vi "TankDrive.vi"(0 "RobotDriveDevRef":T2={"DevStatus"={"status"=FALSE, "code"=0, "source"=""}, "Motors[]"=[], "Square Inputs"=FALSE, "Max Output"=1.0, "Isochronous"=FALSE}, 1 "Action":T1, 5 "Left Motor Value":dbl, 7 "Right Motor Value":dbl, 9 "HalfSpeed":bool=TRUE, 11 "Error In (no error)":errorcluster) -> (15 "Error Out":errorcluster)   [LabVIEW 2013]
doc: "Sets tank drive inputs based on the given action. \nActions:\n-Init: sets the motor values to 0. This is the only time the motor reference is needed; it will be saved for future use.\n-SetValue: sets the motor values to the given values."
uses:
  <vilib>/Rock Robotics/WPI/RobotDrive/WPI_RobotDriveDevRef.ctl
  <vilib>/Rock Robotics/WPI/MotorControl/WPI_MotorControlDeviceRef.ctl
  <vilib>/Rock Robotics/SystemInterfaces/Typedef/FPGA_TypedefDigitalModule.ctl
  <vilib>/Rock Robotics/SystemInterfaces/DIO/FPGA_DIOPWMChannel.ctl
  <vilib>/Rock Robotics/WPI/PWM/WPI_PWMDeadband.ctl
  <vilib>/Rock Robotics/WPI/CAN/Jaguar/SubVIs/WPI_CANJaguar_ControlMode.ctl
  <vilib>/Rock Robotics/WPI/PWM/WPI_PWMTransform_ConPane.ctl
  ActionEnum.ctl
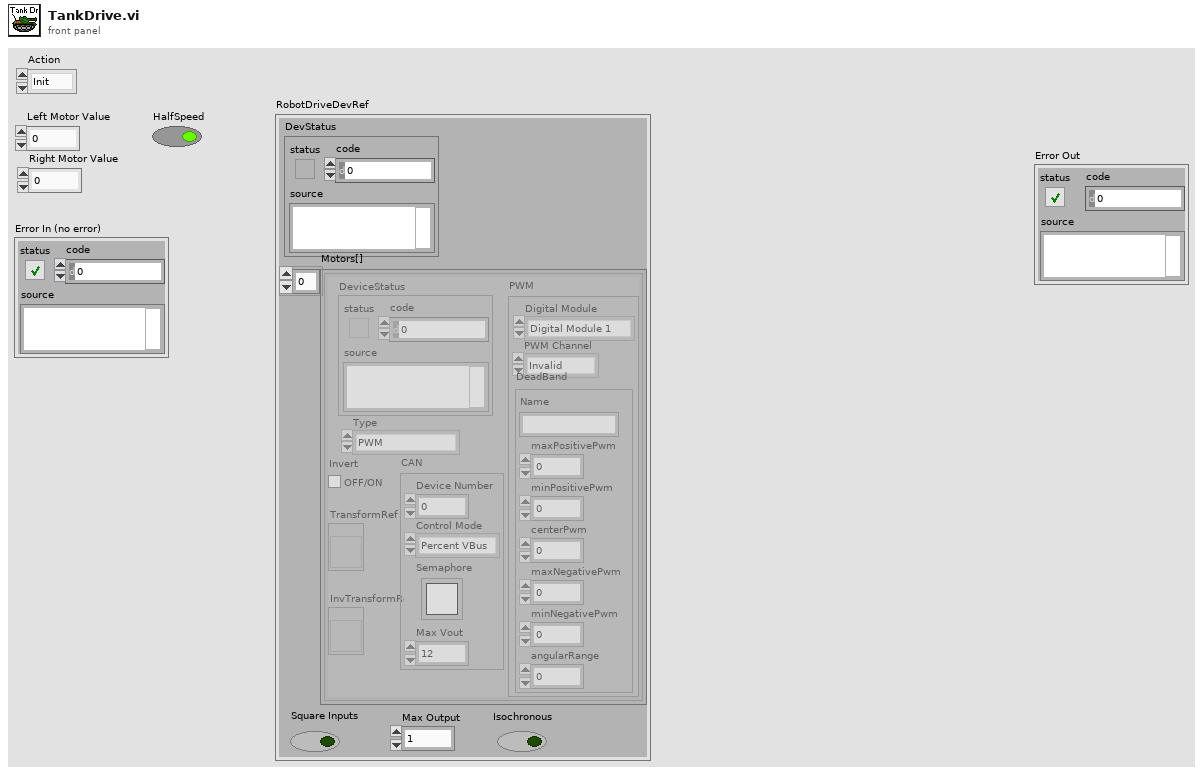
[diagram p1: front panel]
types:
  T1 = typedef "ActionEnum.ctl" = enum16{"Init", "SetValue"}
  T2 = typedef "WPI_RobotDriveDevRef.ctl" = cluster{"DevStatus":errorcluster, "Motors[]":T3[], "Square Inputs":bool, "Max Output":dbl, "Isochronous":bool}
  T3 = typedef "WPI_MotorControlDeviceRef.ctl" = cluster{"DeviceStatus":errorcluster, "Type":enum16{"PWM", "CAN"}, "PWM":cluster{"Digital Module":T4, "PWM Channel":T5, "DeadBand":T6}, "CAN":cluster{"Device Number":u8, "Control Mode":T7, "Semaphore":T8, "Max Vout":dbl}, "Invert":bool, "TransformRef":T9, "InvTransformRef":T9}
  T4 = typedef "FPGA_TypedefDigitalModule.ctl" = enum16{"Digital Module 1", "Digital Module 2"}
  T5 = typedef "FPGA_DIOPWMChannel.ctl" = enum8{"PWM 1", "PWM 2", "PWM 3", "PWM 4", "PWM 5", "PWM 6", "PWM 7", "PWM 8", "PWM 9", "PWM 10", "Invalid"}
  T6 = typedef "WPI_PWMDeadband.ctl" = cluster{"Name":string, "maxPositivePwm":i32, "minPositivePwm":i32, "centerPwm":i32, "maxNegativePwm":i32, "minNegativePwm":i32, "angularRange":u16}
  T7 = typedef "WPI_CANJaguar_ControlMode.ctl" = enum8{"Percent VBus", "Current", "Speed", "Position", "Voltage"}
  T8 = typedef "Semaphore RefNum" = refnum<k1>
  T9 = typedef "WPI_PWMTransform_ConPane.ctl" = refnum<vi>
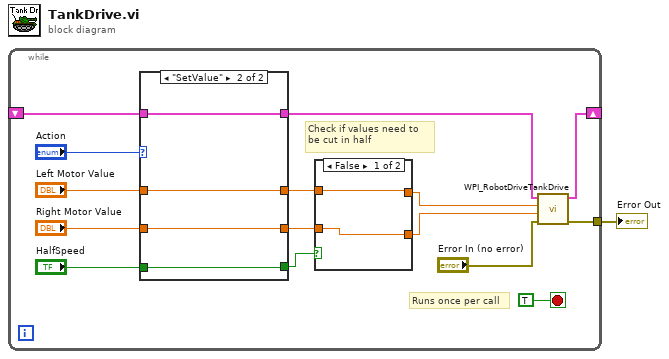
[diagram p0: block diagram]
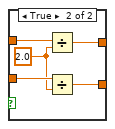
[diagram p2: hidden frame]
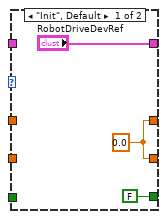
[diagram p3: hidden frame]
diagram:
  n1 = while {
    tunnel: [w15] -> w1
    shift-right: [w3] -> _
    shift-left: _ -> [w4]
    stop <- TRUE stop-if-true
    # "Check if values need to \nbe cut in half"
    # "Runs once per call"
    n2 = case shown="\"SetValue\"" "Action" {
      tunnel: "HalfSpeed" -> [_ w27]
      tunnel: [FALSE w27] -> w10
      tunnel: [w26 w28] -> w8
      tunnel: "Right Motor Value" -> [_ w28]
      tunnel: "Left Motor Value" -> [_ w29]
      tunnel: [w26 w29] -> w6
      tunnel: ["RobotDriveDevRef" w30] -> w5
      tunnel: w4 -> [_ w30]
      frame "Init", Default {
        w26 = 0.0
      }
      frame "SetValue" {
      }
    }
    n3 = case shown="False" w10 {
      tunnel: w8 -> [w18 w22]
      tunnel: w6 -> [w17 w23]
      tunnel: [w17 w20] -> w13
      tunnel: [w18 w19] -> w12
      frame False {
      }
      frame True {
        w21 = 2.0
        n4 = Divide(x=w23, y=w21) -> (x/y=w20:dbl)
        n5 = Divide(x=w22, y=w21) -> (x/y=w19:dbl)
      }
    }
    n6 = call <vilib>:"WPI_RobotDriveTankDrive.vi"("error in (no error)"="Error In (no error)", "Right axis value"=w12, "Left axis value"=w13, "RobotDriveDevRef"=w5) -> ("error out"=w15:errorcluster, "RobotDriveDevRef"=w3:T2)  [unwired: 5 in, 1 out]
  }
  "Error Out" <- w1
